vi "Write BG Color.vi"(8 "error in (no error)":errorcluster, 10 "BG Color":u32(colorbox), 11 "Color Message in":refnum<class "Color Message.lvclass">) -> (0 "error out":errorcluster, 3 "Color Message out":refnum<class "Color Message.lvclass">)   [LabVIEW 2020, in "Color Message.lvclass"]
uses:
  Color Message.lvclass
  Color Message.lvclass/Color Message.ctl
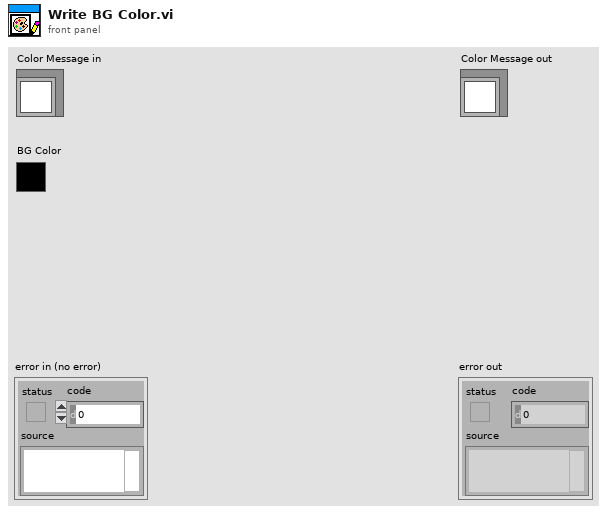
[diagram p1: front panel]
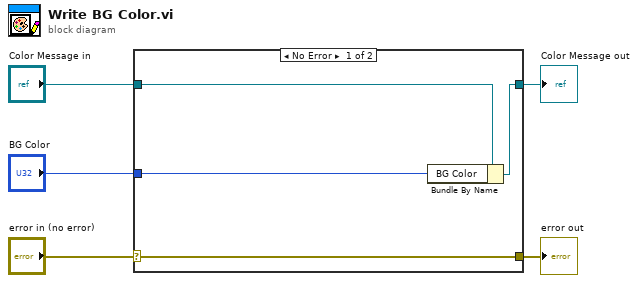
[diagram p0: block diagram]
diagram:
  n1 = case shown="No Error" "error in (no error)" {
    selector: "error in (no error)" -> [w9 w10]
    tunnel: [w9 w10] -> w4
    tunnel: [w7 w11] -> w2
    tunnel: "Color Message in" -> [w8 w11]
    tunnel: "BG Color" -> [w6 _]
    frame No Error {
      n2 = Bundle By Name(cluster=w8, "BG Color"=w6) -> (w7:refnum<class "Color Message.lvclass">)
    }
    frame Error {
    }
  }
  "error out" <- w4
  "Color Message out" <- w2
